vi "GetDeviceName.vi"(11 "Seperator (e.g. \"Channel1\")":string) -> (3 "String":string)   [LabVIEW 2020]
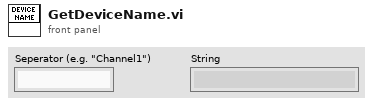
[diagram p1: front panel]
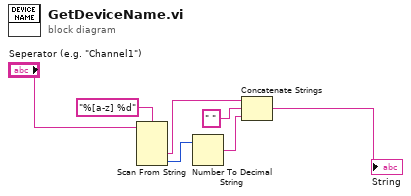
[diagram p0: block diagram]
diagram:
  n1 = Scan From String(format string="%[a-z] %d", input string="Seperator (e.g. \"Channel1\")") -> (output 1=w6:string, output 2=w2:i32)  [unwired: 4 in, 3 out]
  n2 = Number To Decimal String(number=w2) -> (decimal integer string=w4:string)  [unwired: 1 in]
  n3 = Concatenate Strings(w6, " " ("string"), w4) -> (→"String":string)
